vi "22-1.vi"() -> ()   [LabVIEW 2019, in "22.lvlib"]
uses:
  22.lvlib
  Cubes/Cubes.lvclass
  Cube/Cube.lvclass
panel:
  out "Sample Cubes":i64
  out "N Cubes":i64
  in  "Sample Index":i32
  in  "Sample?":bool
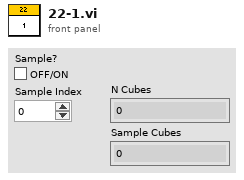
[diagram p1: front panel]
types:
  T1 = cluster{"state":bool, "xmin":i64, "xmax":i64, "ymin":i64, "ymax":i64, "zmin":i64, "zmax":i64}
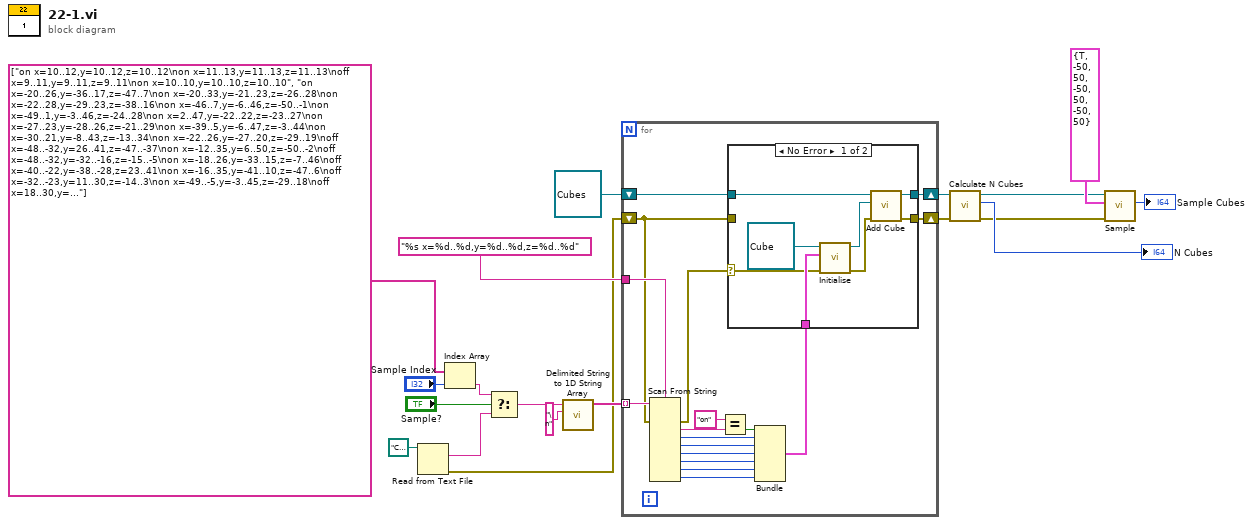
[diagram p0: block diagram]
diagram:
  n1 = Read from Text File(file (use dialog)=path "C:/Users/craig.walker/Documents/GitHub/lv2019-Advent-of-Code-2021/22/input.txt") -> (text=w11:string, error out=w8:errorcluster)  [unwired: 3 in, 2 out]
  n2 = Index Array(array=string[] ["on x=10..12,y=10..12,z=10..12\non x=11..13,y=11..13,z=11..13\noff x=9..11,y=9..11,z=9..11\non x=10..10,y=10..10,z=10..10", "on x=-20..26,y=-36..17,z=-47..7\non x=-20..33,y=-21..23,z=-26..28\non x=-22..28,y=-29..23,z=-38..16\non x=-46..7,y=-6..46,z=-50..-1\non x=-49..1,y=-3..46,z=-24..28\non x=2..47,y=-22..22,z=-23..27\non x=-27..23,y=-28..26,z=-21..29\non x=-39..5,y=-6..47,z=-3..44\non x=-30..21,y=-8..43,z=-13..34\non x=-22..26,y=-27..20,z=-29..19\noff x=-48..-32,y=26..41,z=-47..-37\non x=-12..35,y=6..50,z=-50..-2\noff x=-48..-32,y=-32..-16,z=-15..-5\non x=-18..26,y=-33..15,z=-7..46\noff x=-40..-22,y=-38..-28,z=23..41\non x=-16..35,y=-41..10,z=-47..6\noff x=-32..-23,y=11..30,z=-14..3\non x=-49..-5,y=-3..45,z=-29..18\noff x=18..30,y=-20..-8,z=-3..13\non x=-41..9,y=-7..43,z=-33..15\non x=-54112..-39298,y=-85059..-49293,z=-27449..7877\non x=967..23432,y=45373..81175,z=27513..53682"], index="Sample Index") -> (element=w13:string)
  n3 = Select(t=w13, s="Sample?", f=w11) -> (s? t:f=w15:string)
  n4 = call <vilib>:"Delimited String to 1D String Array.vi"("delimiter"="\n", "delimited string"=w15) -> ("string array"=w17:string[])  [unwired: 9 in]
  n5 = for {
    tunnel: "%s x=%d..%d,y=%d..%d,z=%d..%d" -> [w36]
    tunnel: w17 -> [w35] mode=indexing
    shift-right: [w22] -> w2
    shift-left: refnum<class "Cubes.lvclass"> refnum ("22.lvlib:Cubes.lvclass") -> [w24]
    shift-right: [w21] -> w1
    shift-left: w8 -> [w20]
    n6 = Scan From String(format string=w36, input string=w35, error in=w20) -> (error out=w23:errorcluster, output 1=w34:string, output 2=w31:i32, output 3=w30:i32, output 4=w29:i32, output 5=w28:i32, output 6=w27:i32, output 7=w26:i32)  [unwired: 8 in, 2 out]
    n7 = Equal?(x="on", y=w34) -> (x = y?=w25:bool)
    n8 = Bundle(w25, w31, w30, w29, w28, w27, w26) -> (w32:cluster{bool, i32, i32, i32, i32, i32, i32})  [unwired: 1 in]
    n9 = case shown="No Error" w23 {
      selector: w23 -> [w41 _]
      tunnel: w32 -> [w44 _]
      tunnel: w24 -> [w43 w46]
      tunnel: [w38 w46] -> w22
      tunnel: [w37 w45] -> w21
      tunnel: w20 -> [_ w45]
      frame No Error {
        n10 = call-dynamic "Initialise.vi"("error in (no error)"=w41, "Init"=w44, "Cube in"=refnum<class "Cube.lvclass"> refnum ("22.lvlib:Cube.lvclass")) -> ("error out"=w40:errorcluster, "Cube out"=w42:refnum<class "Cube.lvclass">)  [unwired: 7 in]
        n11 = call-dynamic "Add Cube.vi"("error in (no error)"=w40, "Cube"=w42, "Cubes in"=w43) -> ("error out"=w37:errorcluster, "Cubes out"=w38:refnum<class "Cubes.lvclass">)  [unwired: 7 in]
      }
      frame Error {
      }
    }
  }
  n12 = call-dynamic "Calculate N Cubes.vi"("error in (no error)"=w1, "Cubes in"=w2) -> ("error out"=w4:errorcluster, "N Cubes"=→"N Cubes":i64, "Cubes out"=w3:refnum<class "Cubes.lvclass">)  [unwired: 7 in]
  n13 = call-dynamic "Sample.vi"("error in (no error)"=w4, "Sample Dimensions"=T1 {"state"=TRUE, "xmin"=-50, "xmax"=50, "ymin"=-50, "ymax"=50, "zmin"=-50, "zmax"=50}, "Cubes in"=w3) -> ("N Cubes"=→"Sample Cubes":i64)  [unwired: 6 in, 2 out]
